vi "test-trajectory-concatenate.vi"(8 "error in (no error)":errorcluster) -> (0 "error out":errorcluster, 3 "TEsts Passed":bool)   [LabVIEW 2019]
uses:
  <vilib>/Rock Robotics/WPI/ThirdParty/JAS_Junk/TrajLib/TRAJECTORY.ctl
  <vilib>/Rock Robotics/WPI/ThirdParty/JAS_Junk/TrajLib/TRAJ_STATE.ctl
  <vilib>/Rock Robotics/WPI/ThirdParty/JAS_Junk/TrajLib/POSE2D.ctl
  <vilib>/Rock Robotics/WPI/ThirdParty/JAS_Junk/TrajLib/TRANSLATION2D.ctl
  <vilib>/Rock Robotics/WPI/ThirdParty/JAS_Junk/TrajLib/ROTATION2D.ctl
  <vilib>/Rock Robotics/WPI/ThirdParty/JAS_Junk/TrajLib/TRAJECTORY_SPLINE_TYPE_ENUM.ctl
  <vilib>/Rock Robotics/WPI/ThirdParty/JAS_Junk/TrajLib/Translation2d_Create.vi
  <vilib>/Rock Robotics/WPI/ThirdParty/JAS_Junk/TrajLib/Rotation2d_CreateAngle.vi
  <vilib>/Rock Robotics/WPI/ThirdParty/JAS_Junk/TrajLib/Translation2d_Equals.vi
  <vilib>/Rock Robotics/WPI/ThirdParty/JAS_Junk/TrajLib/Rotation2d_Equals.vi
  <vilib>/Rock Robotics/WPI/ThirdParty/JAS_Junk/TrajLib/Util_CalcDist.vi
  <vilib>/Rock Robotics/WPI/ThirdParty/JAS_Junk/TrajLib/Trajectory_Library.lvlib
panel:
  out "AddTimes":dbl
  out "concat Traj":T1 {"States"."POSE"."ROTATION"."SIN" format="%13.4f"; "States"."POSE"."ROTATION"."COS" format="%13.4f"; "States"."POSE"."ROTATION"."VALUE" format="%13.4f"; "States"."POSE"."TRANSLATION"."Y" format="%14.3f"; "States"."POSE"."TRANSLATION"."X" format="%14.3f"; "TotalTImeSecs" format="%20.3f"}
  out "Problem":bool
  out "TotalTime_Sec":dbl
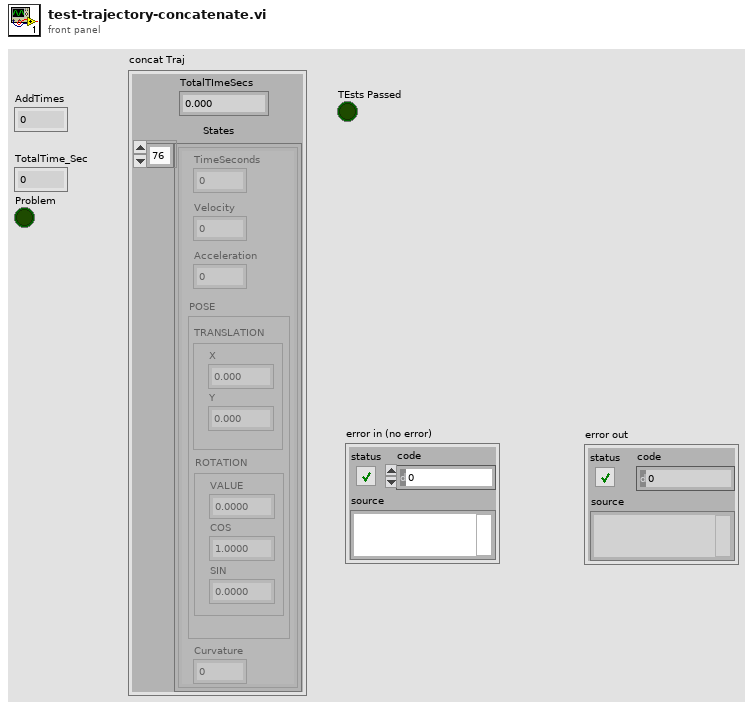
[diagram p1: front panel]
types:
  T1 = typedef "Trajectory_Library.lvlib/TRAJECTORY.ctl" = cluster{"TotalTImeSecs":dbl, "States":T2[]}
  T2 = typedef "Trajectory_Library.lvlib/TRAJ_STATE.ctl" = cluster{"TimeSeconds":dbl, "Velocity":dbl, "Acceleration":dbl, "POSE":T3, "Curvature":dbl}
  T3 = typedef "Trajectory_Library.lvlib/POSE2D.ctl" = cluster{"TRANSLATION":T4, "ROTATION":T5}
  T4 = typedef "Trajectory_Library.lvlib/TRANSLATION2D.ctl" = cluster{"X":dbl, "Y":dbl}
  T5 = typedef "Trajectory_Library.lvlib/ROTATION2D.ctl" = cluster{"VALUE":dbl, "COS":dbl, "SIN":dbl}
  T6 = typedef "Trajectory_Library.lvlib/TRAJECTORY_SPLINE_TYPE_ENUM.ctl" = enum16{"Cubic", "Cubic With Weights", "Quintic", "Quintic With Weights"}
  T7 = typedef "Trajectory_Library.lvlib/TRAJ_CONFIG.ctl" = cluster{"MaxVelocity":dbl, "Max Acceleration":dbl, "StartVelocity":dbl, "End Velocity":dbl, "Reversed":bool, "DiffDrKineConstntDefined":bool, "CentAcellConstntDefined":bool, "DiffDrVoltConstntDefined":bool, "DIFF_DRIVE_KINE_CONSTRAINT":T8, "CENTRIPETAL_ACCEL_CONSTRAINT":T10, "SwerveDrKineConstntDefined":bool, "SWERVE_DRIVE_KINE_CONSTRAINT":T11, "DIFF_DRIVE_VOLTAGE_CONSTRAINT":T14, "MECANUM_DRIVE_KINE_CONSTRAINT":T16, "MecanumDrKineConstntDefined":bool}
  T8 = typedef "Trajectory_Library.lvlib/TRAJ_CONSTRAINT_DIIF_DRIVE_KINEMATICS.ctl" = cluster{"Max Speed (M/S)":dbl, "DIFF_DRIVE_KINEMATICS":T9, "Max Accel (M/S2)":dbl}
  T9 = typedef "Trajectory_Library.lvlib/DIFF_DRIVE_KINEMATICS.ctl" = cluster{"TrackWidth_Meters":dbl}
  T10 = typedef "Trajectory_Library.lvlib/TRAJ_CONSTRAINT_CENTRIPETAL_ACCEL.ctl" = cluster{"Max Cent Accel":dbl}
  T11 = typedef "Trajectory_Library.lvlib/TRAJ_CONSTRAINT_SWERVE_DRIVE_KINEMATICS.ctl" = cluster{"Max Speed (M/S)":dbl, "SwerveKinematics":T12}
  T12 = typedef "Trajectory_Library.lvlib/SWERVE_DRIVE_KINEMATICS.ctl" = cluster{"NumModules":i32, "InverseKinematics":T13, "ForwardKinematics":T13, "Modules":T4[], "PrevCoR":T4}
  T13 = typedef "NI_Matrix.lvlib/RealMatrix.ctl" = dbl[][]
  T14 = typedef "Trajectory_Library.lvlib/TRAJ_CONSTRAINT_DIIF_DRIVE_VOLTAGE.ctl" = cluster{"Max Voltage":dbl, "DIFF_DRIVE_KINEMATICS":T9, "SIMPLE_MOTOR_FF":T15}
  T15 = typedef "Trajectory_Library.lvlib/SIMPLE_MOTOR_FF.ctl" = cluster{"Ks":dbl, "Kv":dbl, "Ka":dbl}
  T16 = typedef "Trajectory_Library.lvlib/TRAJ_CONSTRAINT_MECA_DRIVE_KINEMATICS.ctl" = cluster{"Max Speed (M/S)":dbl, "MECA_DRIVE_KINEMATICS":T17}
  T17 = typedef "Trajectory_Library.lvlib/MECA_DRIVE_KINEMATICS.ctl" = cluster{"FrontLeft":T4, "FrontRight":T4, "RearLeft":T4, "RearRight":T4, "InverseKinematics":T13, "ForwardKinematics":T13, "PrevCoR":T4}
  T18 = typedef "Trajectory_Library.lvlib/WEIGHTED_WAYPOINT.ctl" = cluster{"TRANSLATION":T4, "ROTATION":T5, "SCALAR":dbl}
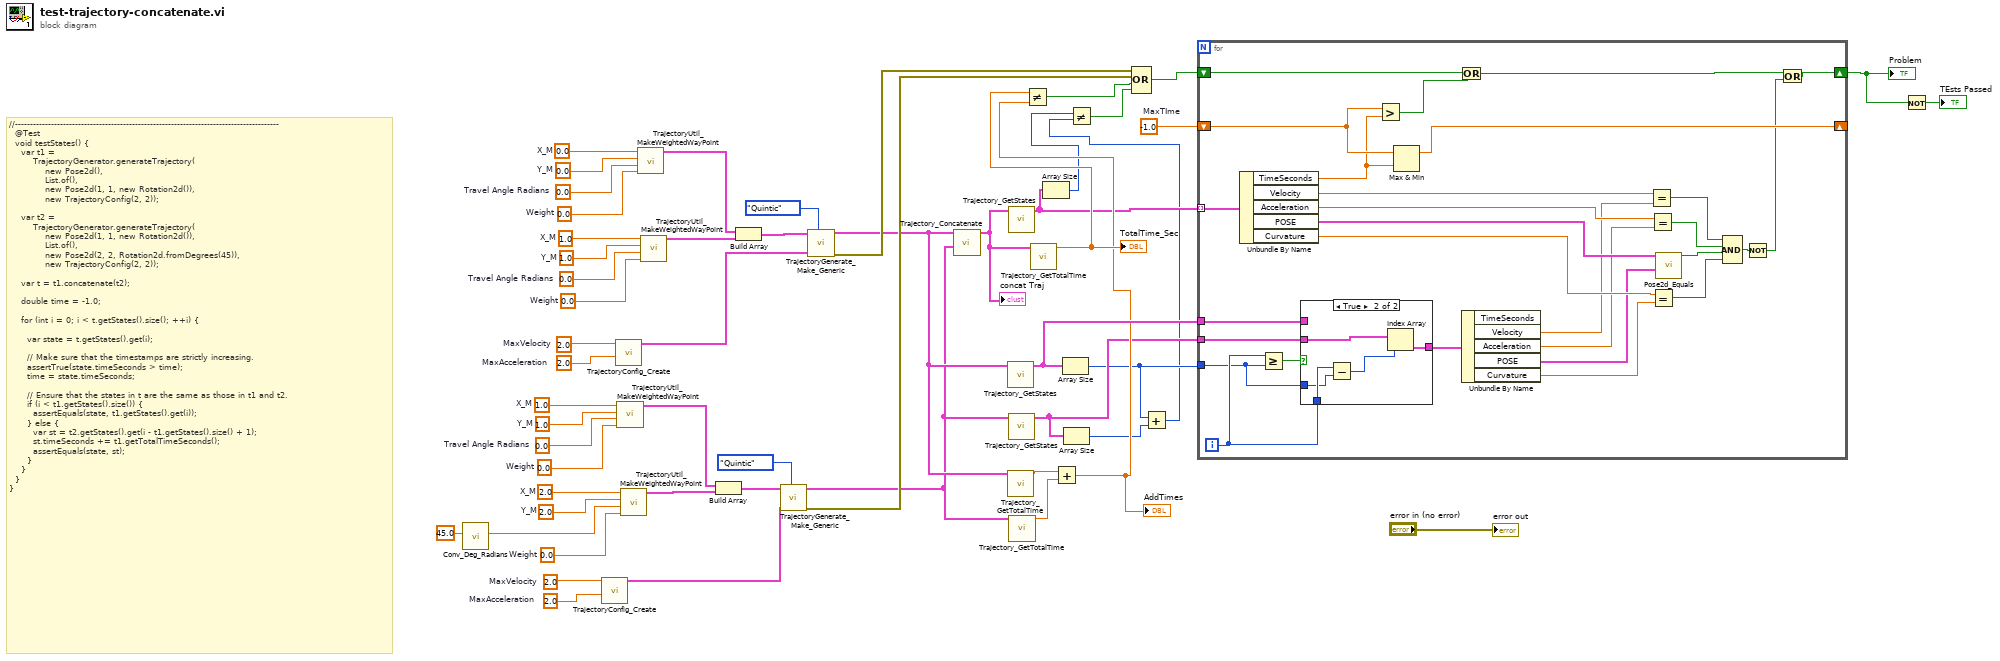
[diagram p0: block diagram]
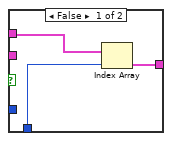
[diagram p2: hidden frame]
diagram:
  w20 = -1.0  # MaxTIme
  w38 = 2.0  # X_M
  w37 = 2.0  # Y_M
  w36 = 0.0  # Weight
  w35 = 1.0  # X_M
  w34 = 1.0  # Y_M
  w33 = 0.0  # Travel Angle Radians
  w32 = 0.0  # Weight
  w31 = 2.0  # MaxVelocity
  w30 = 2.0  # MaxAcceleration
  w53 = 1.0  # X_M
  w52 = 1.0  # Y_M
  w51 = 0.0  # Travel Angle Radians
  w50 = 0.0  # Weight
  w49 = 0.0  # X_M
  w48 = 0.0  # Y_M
  w47 = 0.0  # Travel Angle Radians
  w46 = 0.0  # Weight
  w45 = 2.0  # MaxVelocity
  w44 = 2.0  # MaxAcceleration
  # "//----------------------------------------------------------------------------------------\n  @Test\n  void testStates() {\n    var t1 =\n        TrajectoryGenerator.generateTrajectory(\n            new Pose2d(),\n            List.of(),\n            new Pose2d(1, 1, new Rotation2d()),\n            new TrajectoryConfig(2, 2));\n\n    var t2 =\n        TrajectoryGenerator.generateTrajectory(\n            new Pose2d(1, 1, new Rotation2d()),\n            List.of(),\n            new Pose2d(2, 2, Rotation2d.fromDegrees(45)),\n            new TrajectoryConfig(2, 2));\n\n    var t = t1.concatenate(t2);\n\n    double time = -1.0;\n\n    for (int i = 0; i < t.getStates().size(); ++i) {\n\n      var state = t.getStates().get(i);\n\n      // Make sure that the timestamps are strictly increasing.\n      assertTrue(state.timeSeconds > time);\n      time = state.timeSeconds;\n\n      // Ensure that the states in t are the same as those in t1 and t2.\n      if (i < t1.getStates().size()) {\n        assertEquals(state, t1.getStates().get(i));\n      } else {\n        var st = t2.getStates().get(i - t1.getStates().size() + 1);\n        st.timeSeconds += t1.getTotalTimeSeconds();\n        assertEquals(state, st);\n      }\n    }\n  }\n}"
  n1 = call <vilib>:"Conv_Deg_Radians.vi"("Degress"=45.0) -> ("Radians"=w24:dbl)  [unwired: 10 in]
  n2 = call <vilib>:"TrajectoryConfig_Create.vi"("MaxAcceleration"=w30, "MaxVelocity"=w31) -> ("TRAJECTORY_CONFIG"=w29:T7)  [unwired: 9 in]
  n3 = call <vilib>:"TrajectoryConfig_Create.vi"("MaxAcceleration"=w44, "MaxVelocity"=w45) -> ("TRAJECTORY_CONFIG"=w43:T7)  [unwired: 9 in]
  n4 = call <vilib>:"TrajectoryUtil_MakeWeightedWayPoint.vi"("Weight"=w32, "Travel Angle Radians"=w33, "Y_M"=w34, "X_M"=w35) -> ("WEIGHTED_WAYPOINT"=w26:T18)  [unwired: 7 in]
  n5 = call <vilib>:"TrajectoryUtil_MakeWeightedWayPoint.vi"("Weight"=w36, "Travel Angle Radians"=w24, "Y_M"=w37, "X_M"=w38) -> ("WEIGHTED_WAYPOINT"=w39:T18)  [unwired: 7 in]
  n6 = call <vilib>:"TrajectoryUtil_MakeWeightedWayPoint.vi"("Weight"=w46, "Travel Angle Radians"=w47, "Y_M"=w48, "X_M"=w49) -> ("WEIGHTED_WAYPOINT"=w40:T18)  [unwired: 7 in]
  n7 = call <vilib>:"TrajectoryUtil_MakeWeightedWayPoint.vi"("Weight"=w50, "Travel Angle Radians"=w51, "Y_M"=w52, "X_M"=w53) -> ("WEIGHTED_WAYPOINT"=w54:T18)  [unwired: 7 in]
  n8 = Build Array(w26, w39) -> (w27:T18[])
  n9 = Build Array(w40, w54) -> (w41:T18[])
  n10 = call <vilib>:"TrajectoryGenerate_Make_Generic.vi"("Spline Type"=TRAJECTORY_SPLINE_TYPE_ENUM."Quintic", "traj_config"=w29, "WeightedWayPoints"=w27) -> ("error out"=w22:errorcluster, "TRAJECTORY"=w16:T1)  [unwired: 7 in]
  n11 = call <vilib>:"TrajectoryGenerate_Make_Generic.vi"("Spline Type"=TRAJECTORY_SPLINE_TYPE_ENUM."Quintic", "traj_config"=w43, "WeightedWayPoints"=w41) -> ("error out"=w23:errorcluster, "TRAJECTORY"=w17:T1)  [unwired: 7 in]
  n12 = call <vilib>:"Trajectory_Concatenate.vi"("InputTRAJECTORY 2"=w16, "InputTRAJECTORY"=w17) -> ("outputTRAJECTORY"=w21:T1)  [unwired: 9 in]
  "concat Traj" <- w21
  n13 = call <vilib>:"Trajectory_GetStates.vi"("TRAJECTORY"=w17) -> ("States"=w18:T2[])  [unwired: 10 in]
  n14 = call <vilib>:"Trajectory_GetTotalTime.vi"("TRAJECTORY"=w17) -> ("TotalTime_Sec"=w15:dbl)  [unwired: 10 in]
  n15 = call <vilib>:"Trajectory_GetStates.vi"("TRAJECTORY"=w21) -> ("States"=w10:T2[])  [unwired: 10 in]
  n16 = call <vilib>:"Trajectory_GetStates.vi"("TRAJECTORY"=w16) -> ("States"=w9:T2[])  [unwired: 10 in]
  n17 = call <vilib>:"Trajectory_GetTotalTime.vi"("TRAJECTORY"=w16) -> ("TotalTime_Sec"=w14:dbl)  [unwired: 10 in]
  n18 = call <vilib>:"Trajectory_GetTotalTime.vi"("TRAJECTORY"=w21) -> ("TotalTime_Sec"=w12:dbl)  [unwired: 10 in]
  "TotalTime_Sec" <- w12
  n19 = Array Size(array=w10) -> (size(s)=w6:i32)
  n20 = Add(x=w15, y=w14) -> (x+y=w11:dbl)
  "AddTimes" <- w11
  n21 = Not Equal?(x=w12, y=w11) -> (x != y?=w13:bool)
  n22 = Array Size(array=w18) -> (size(s)=w7:i32)
  n23 = Array Size(array=w9) -> (size(s)=w8:i32)
  n24 = Add(x=w7, y=w8) -> (x+y=w5:i32)
  n25 = Not Equal?(x=w6, y=w5) -> (x != y?=w4:bool)
  n26 = Compound Arithmetic op=OR(w23, w22, w13, w4) -> (w19:bool)
  n27 = for {
    tunnel: w10 -> [w82] mode=indexing
    shift-right: [w57] -> w3
    shift-left: w19 -> [w78]
    shift-right: [w77] -> _
    shift-left: w20 -> [w81]
    tunnel: w7 -> [w73]
    tunnel: w18 -> [w76]
    tunnel: w9 -> [w74]
    i -> [w75]
    n28 = Unbundle By Name(w82) -> ("TimeSeconds"=w80:dbl, "Velocity"=w71:dbl, "Acceleration"=w70:dbl, "POSE"=w69:T3, "Curvature"=w68:dbl)
    n29 = Greater Or Equal?(x=w75, y=w73) -> (x >= y?=w55:bool)
    n30 = case shown="True" w55 {
      tunnel: w76 -> [w85 _]
      tunnel: w75 -> [w84 w88]
      tunnel: [w83 w86] -> w72
      tunnel: w74 -> [_ w90]
      tunnel: w73 -> [_ w87]
      frame False {
        n31 = Index Array(array=w85, index=w84) -> (element=w83:T2)
      }
      frame True {
        n32 = Subtract(x=w88, y=w87) -> (x-y=w89:i32)
        n33 = Index Array(array=w90, index=w89) -> (element=w86:T2)
      }
    }
    n34 = Greater?(x=w81, y=w80) -> (0:w79:bool)
    n35 = Max & Min(x=w81, y=w80) -> (max(x,y)=w77:dbl)  [unwired: 1 out]
    n36 = Or(x=w78, y=w79) -> (x .or. y?=w56:bool)
    n37 = Unbundle By Name(w72) -> ("Velocity"=w67:dbl, "Acceleration"=w65:dbl, "POSE"=w66:T3, "Curvature"=w64:dbl)  [unwired: 1 out]
    n38 = Equal?(x=w71, y=w67) -> (x = y?=w63:bool)
    n39 = Equal?(x=w70, y=w65) -> (x = y?=w62:bool)
    n40 = Equal?(x=w68, y=w64) -> (x = y?=w60:bool)
    n41 = call <vilib>:"Pose2d_Equals.vi"("other POSE"=w66, "in POSE"=w69) -> ("Equals"=w61:bool)  [unwired: 9 in]
    n42 = Compound Arithmetic op=AND(w63, w62, w61, w60) -> (w59:bool)
    n43 = Not(x=w59) -> (.not. x?=w58:bool)
    n44 = Or(x=w56, y=w58) -> (x .or. y?=w57:bool)
  }
  "Problem" <- w3
  n45 = Not(x=w3) -> (.not. x?=→"TEsts Passed":bool)
  "error out" <- "error in (no error)"
